vi "Utility Check Options.vi"(8 "error in (no error)":errorcluster {"code" format="%.0x"}, 10 "Search Options":string, 11 "VISA Resource Name":refnum<visa-resource-name>) -> (0 "error out":errorcluster {"code" format="%.0x"}, 2 "Found":bool, 3 "VISA Resource Name Out":refnum<visa-resource-name>)   [LabVIEW 2014, in "Agilent ESG Series.lvlib"]
doc: "This utility VI reads options that are installed in the intrument."
uses:
  Agilent ESG Series.lvlib
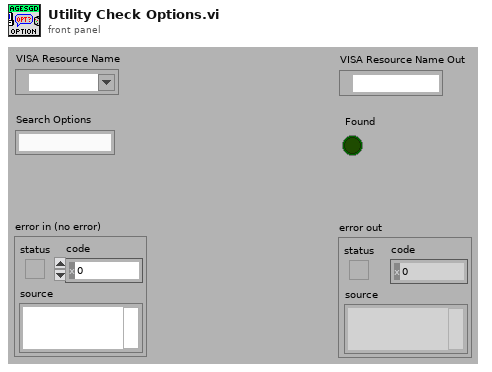
[diagram p1: front panel]
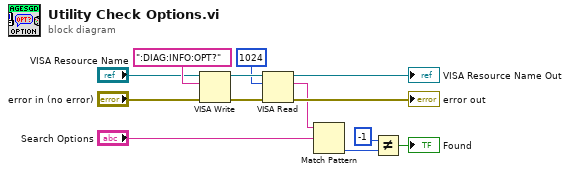
[diagram p0: block diagram]
diagram:
  n1 = VISA Write(VISA resource name="VISA Resource Name", write buffer=":DIAG:INFO:OPT?", error in (no error)="error in (no error)") -> (VISA resource name out=w11:refnum<visa-resource-name>, error out=w10:errorcluster)  [unwired: 1 out]
  n2 = VISA Read(VISA resource name=w11, byte count=u32 1024, error in (no error)=w10) -> (VISA resource name out=→"VISA Resource Name Out":refnum<visa-resource-name>, read buffer=w4:string, error out=→"error out":errorcluster)  [unwired: 1 out]
  n3 = Match Pattern(string=w4, regular expression="Search Options") -> (offset past match=w3:i32)  [unwired: 1 in, 3 out]
  n4 = Not Equal?(x=-1, y=w3) -> (x != y?=→"Found":bool)
